vi "Terminate Session.vi"(8 "error in (no error)":errorcluster, 10 "Destroy (T)":bool=TRUE, 11 "Session in":refnum<class "Session.lvclass">) -> (0 "error out":errorcluster, 2 "Destroyed":bool, 3 "Session out":refnum<class "Session.lvclass">)   [LabVIEW 2013, in "MQTT Base.lvlib" / "Session.lvclass"]
doc: "Set the \"Destroy\" flag to True if the Connection Handler terminates to force the session to be destroyed for good, no matter what the CleanSession flag state is.\nIf the Connection Handler does not terminate and the CleanSession flag is false, then the Session's process stops but the last state of the session is maintained for a possible client reconnection."
uses:
  Session.lvclass
  Session.lvclass/Session.ctl
  MQTT_Connection/Connection/Connection.lvclass
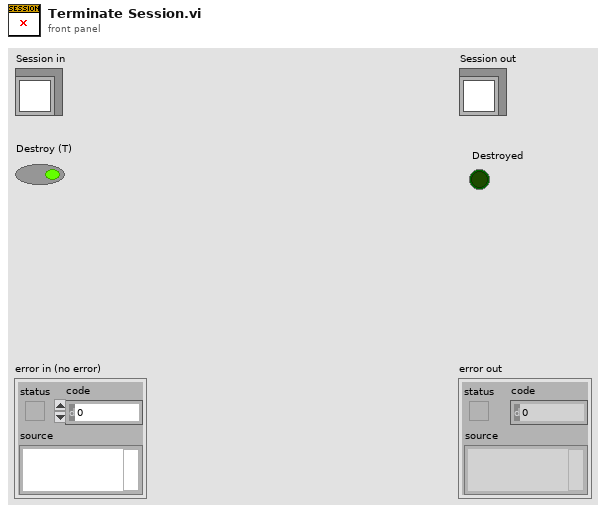
[diagram p1: front panel]
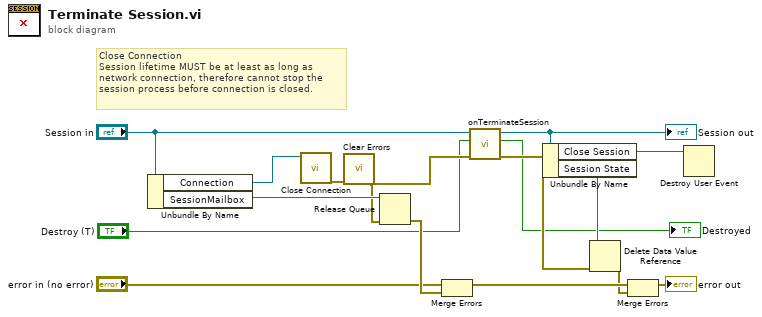
[diagram p0: block diagram]
diagram:
  # "Close Connection\nSession lifetime MUST be at least as long as \nnetwork connection, therefore cannot stop the\nsession process before connection is closed."
  n1 = Unbundle By Name("Session in") -> ("Connection"=w15:refnum<class "Connection.lvclass">, "SessionMailbox"=w16:refnum<queue>)
  n2 = call "Close Connection.vi"("Connection in"=w15) -> ("error out"=w14:errorcluster)  [unwired: 9 in, 1 out]
  n3 = call <vilib>:"Clear Errors.vi"("error in (no error)"=w14) -> ("error out"=w8:errorcluster)  [unwired: 6 in]
  n4 = Release Queue(queue=w16, error in (no error)=w8) -> (error out=w13:errorcluster)  [unwired: 1 in, 2 out]
  n5 = Merge Errors("error in (no error)", w13) -> (w12:errorcluster)
  n6 = call-dynamic "onTerminateSession.vi"("error in (no error)"=w8, "Destroy (T)"="Destroy (T)", "Session in"="Session in") -> ("error out"=w7:errorcluster, "Session Destroyed"=→"Destroyed":bool, "Session out"=w5:refnum<class "Session.lvclass">)  [unwired: 6 in]
  "Session out" <- w5
  n7 = Unbundle By Name(w5) -> ("Close Session"=w1:refnum<user-event>, "Session State"=w9:refnum<data-value>)
  n8 = Delete Data Value Reference(data value reference=w9, error in=w7) -> (error out=w10:errorcluster)  [unwired: 1 out]
  n9 = Merge Errors(w12, w10) -> (→"error out":errorcluster)
  n10 = Destroy User Event(user event=w1) -> ()  [unwired: 1 in, 1 out]
